vi "FlukeTiming.vi"(8 "UTC":i16=-3, 10 "file timestamp":timestamp format="%^<%.3X\n%x>T", 11 "array":string[](array[string])) -> (3 "timestamp out":timestamp format="%^<%.3X\n%x>T")   [LabVIEW 2014]
panel:
  out "extended precision float":ext format="%_14f"
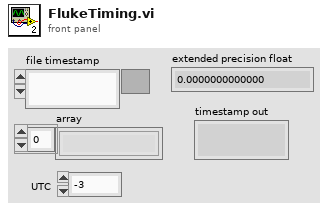
[diagram p1: front panel]
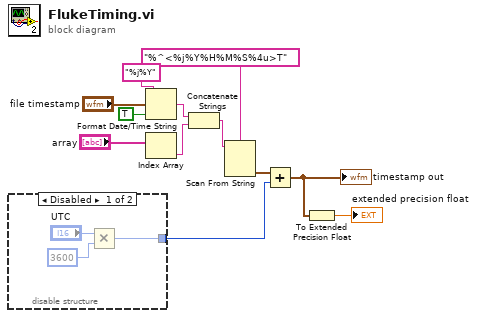
[diagram p0: block diagram]
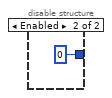
[diagram p2: hidden frame]
diagram:
  n1 = disable-structure shown="Disabled" {
    disable-tunnel: [w13 i16 0] -> w3
    frame Disabled {
      n2 = Multiply(x="UTC", y=i16 3600) -> (x*y=w13:i16)
    }
    frame Enabled {
    }
  }
  n3 = Format Date/Time String(time format string (%c)="%j%Y", seconds (now)="file timestamp", UTC format=TRUE) -> (date/time string=w9:string)
  n4 = Index Array(array="array") -> (element=w11:string)  [unwired: 1 in]
  n5 = Concatenate Strings(w9, w11) -> (w10:string)
  n6 = Scan From String(format string="%^<%j%Y%H%M%S%4u>T", input string=w10) -> (output 1=w4:timestamp)  [unwired: 3 in, 3 out]
  n7 = Add(x=w4, y=w3) -> (x+y=w2:timestamp)
  "timestamp out" <- w2
  n8 = To Extended Precision Float(1:w2) -> (0:→"extended precision float":ext)
